vi "Unit conversion.vi"(4 "Convert to":enum16{"oz.in", "lbf-ft.", "lbf-in.", "N-m"}(ring), 5 "data in":waveform(dbl)={"t0"=timestamp(0 s since 1904-01-01), "dt"=0.0, "Y"=[]}) -> (1 "Unit":string, 2 "Torque":dbl, 3 "waveform out":waveform(dbl)(graph))   [LabVIEW 2018]
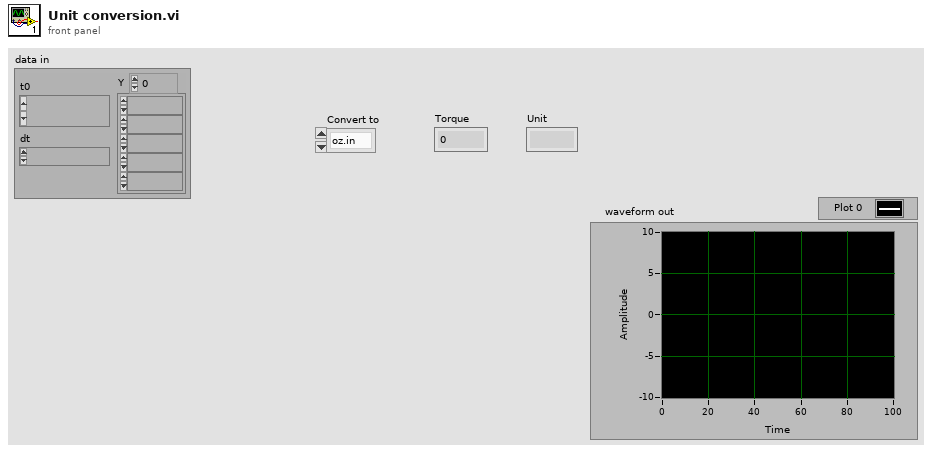
[diagram p1: front panel]
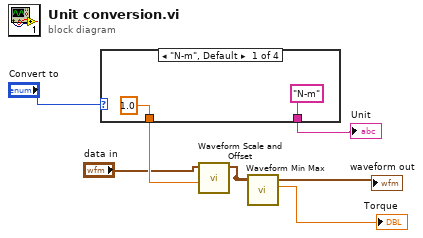
[diagram p0: block diagram]
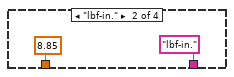
[diagram p2: hidden frame]
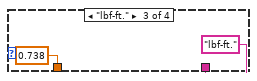
[diagram p3: hidden frame]
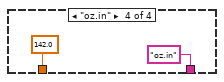
[diagram p4: hidden frame]
diagram:
  n1 = case shown="\"N-m\", Default" "Convert to" {
    tunnel: ["N-m" "lbf-in." "lbf-ft." "oz.in"] -> w5
    tunnel: [1.0 8.85 ("y") 0.738 ("y") 142.0 ("y")] -> w4
    frame "N-m", Default {
    }
    frame "lbf-in." {
    }
    frame "lbf-ft." {
    }
    frame "oz.in" {
    }
  }
  "Unit" <- w5
  n2 = call <vilib>:"Waveform Scale and Offset.vi"("scale"=w4, "waveform in"="data in") -> ("waveform out"=w3:waveform(dbl))  [unwired: 8 in, 1 out]
  "waveform out" <- w3
  n3 = call <vilib>:"Waveform Min Max.vi"("waveform in"=w3) -> ("Y max"=→"Torque":dbl)  [unwired: 5 in, 5 out]
